vi "Plot Pose2d PtbyPt.vi"(7 "Reset? (F)":bool, 10 "dt":dbl, 11 "Pose2d":T1) -> (3 "Pose Telemetry":cluster{dbl[], dbl[]}[](graph))   [LabVIEW 2019]
uses:
  Geometry/Typedef/Pose2d.ctl
  Geometry/Typedef/Translation2d.ctl
  Geometry/Typedef/Rotation2d.ctl
  Typedef/Trajectory State.ctl
  <vilib>/ptbypt/NI_PtbyPt.lvlib
panel:
  out "Waveform Chart 2":dbl(graph)
  out "Waveform Chart":dbl(graph)
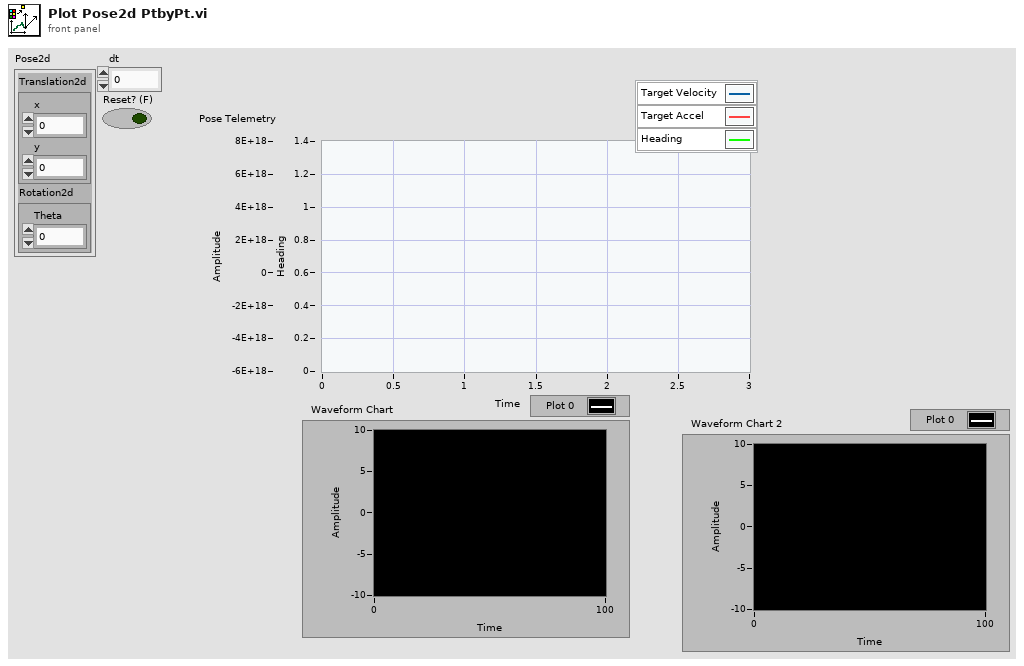
[diagram p1: front panel]
types:
  T1 = typedef "Pose2d.ctl" = cluster{"Translation2d":T2, "Rotation2d":T3}
  T2 = typedef "Translation2d.ctl" = cluster{"x":dbl, "y":dbl}
  T3 = typedef "Rotation2d.ctl" = cluster{"Theta":dbl}
  T4 = typedef "Trajectory State.ctl" = cluster{"t":dbl, "velocity":dbl, "acceleration":dbl, "pose":T1, "curvature":dbl}
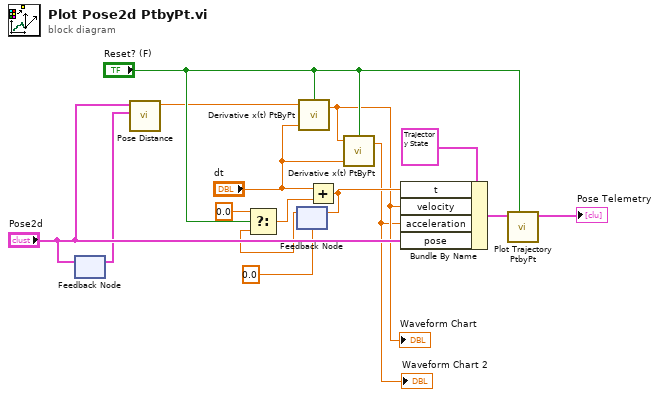
[diagram p0: block diagram]
diagram:
  n1 = feedback-in #1("Pose2d") -> ()
  n2 = feedback #1() -> (w11:T1)  [unwired: 1 in]
  n3 = call "Pose Distance.vi"("Pose2d 2"=w11, "Pose2d"="Pose2d") -> ("Distance"=w3:dbl)  [unwired: 9 in]
  n4 = feedback #2(0.0) -> (w6:dbl)
  n5 = Select(t=0.0, s="Reset? (F)", f=w6) -> (s? t:f=w7:dbl)
  n6 = call <vilib>:"Derivative x(t) PtByPt.vi"("initialize"="Reset? (F)", "dt"="dt", "x"=w3) -> ("dx/dt"=w2:dbl)  [unwired: 1 in, 1 out]
  "Waveform Chart" <- w2
  n7 = Add(x="dt", y=w7) -> (x+y=w9:dbl)
  n8 = feedback-in #2(w9) -> ()
  n9 = call <vilib>:"Derivative x(t) PtByPt.vi"("initialize"="Reset? (F)", "dt"="dt", "x"=w2) -> ("dx/dt"=w1:dbl)  [unwired: 1 in, 1 out]
  "Waveform Chart 2" <- w1
  n10 = Bundle By Name(cluster=T4 {"t"=0.0, "velocity"=0.0, "acceleration"=0.0, "pose"={"Translation2d"={"x"=0.0, "y"=0.0}, "Rotation2d"={"Theta"=0.0}}, "curvature"=0.0} ("State"), "t"=w9, "velocity"=w2, "acceleration"=w1, "pose"="Pose2d") -> (w14:T4)
  n11 = call "Plot Trajectory PtbyPt.vi"("Reset? (F)"="Reset? (F)", "State"=w14) -> ("Telemetry"=→"Pose Telemetry":cluster{dbl[], dbl[]}[])  [unwired: 9 in]
